vi "Export File - Rx Packet XML.vi"(4 "Rx Packet":T2 {"targetPriority" min=-2 max=16 step=1; "targetProcessor" min=-2 max=16 step=1; "Endianness" items=["big-endian"=0, "little-endian"=2]}, 6 "RootNode":refnum<k24>, 8 "error in (no error)":errorcluster, 9 "Rx Packet Header Data":T1, 11 "XmlDocument in":refnum<k24>) -> (0 "error out":errorcluster, 3 "XmlDocument out":refnum<k24>)   [LabVIEW 2019, in "UDP-Custom-Device System Explorer.lvlib"]
uses:
  UDP-Custom-Device System Explorer.lvlib
  System.Xml
  Types/XML - New/ImpExp - Rx Packet Data.ctl
  <vilib>/NI VeriStand/Custom Device API/Custom Device Item Info.ctl
  Shared/Types/Shared - Channel Data Type.ctl
  Shared/Types/Shared - Buffered.PacketInfo.ctl
  Shared/Types/Shared - Pointer Encoding.ctl
  Shared/Types/Shared - Receive Buffer Options.ctl
  Shared/Types/Shared - Transmit Buffer Options.ctl
  Shared/Types/Shared - New Data Options.ctl
  Shared/Types/Shared - Thread Management.ctl
  Types/XML - New/ImpExp - Packet Headers.ctl
  Shared/UDP-Custom-Device Shared.lvlib
  <vilib>/NI VeriStand/Custom Device API/Custom Device API.lvlib
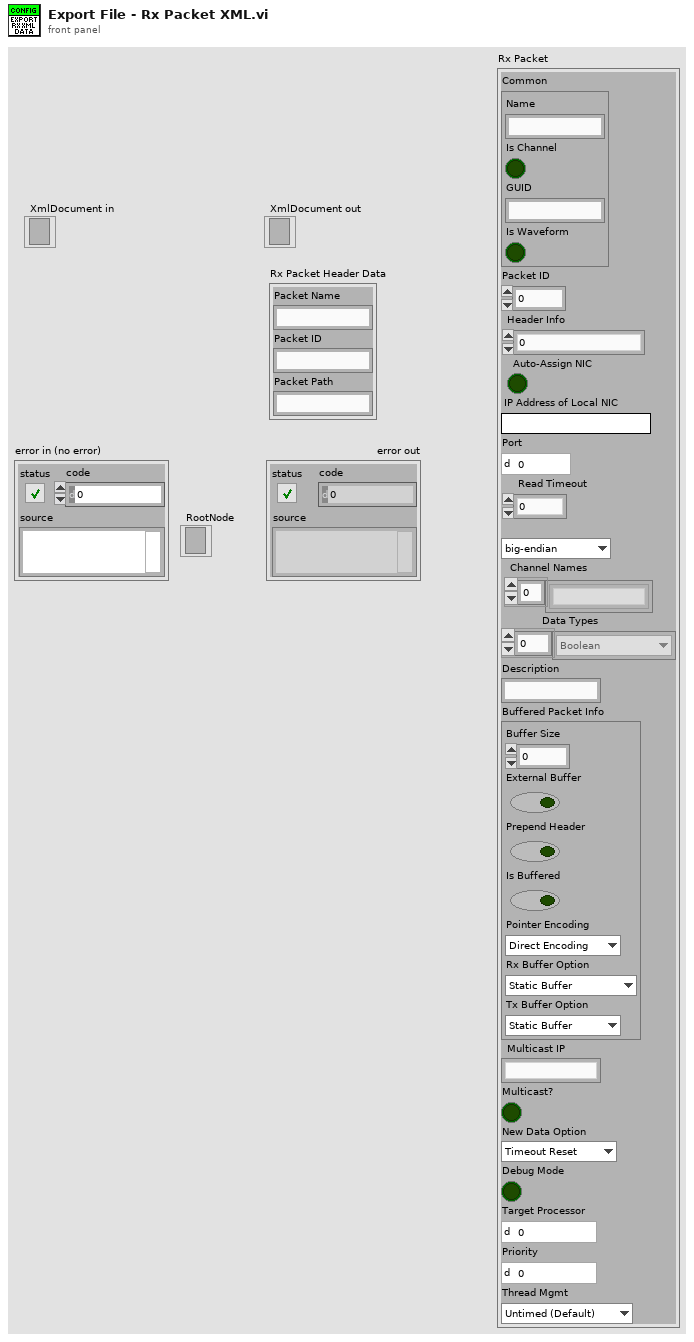
[diagram p1: front panel]
types:
  T1 = typedef "UDP-Custom-Device System Explorer.lvlib/ImpExp - Packet Headers.ctl" = cluster{"Packet Name":string, "Packet ID":string, "Packet Path":string}
  T2 = typedef "UDP-Custom-Device System Explorer.lvlib/ImpExp - Rx Packet Data.ctl" = cluster{"Common":T3, "Packet ID":i32, "Header Info":u32, "Auto-Assign NIC":bool, "IP Address of Local NIC":string, "Port":u16, "Read Timeout":i32, "Endianness":u16, "Channel Names":string[], "Data Types":T4[], "Description":string, "Buffered Packet Info":T5, "Multicast IP":string, "Multicast?":bool, "New Data Option":T9, "Debug Mode":bool, "targetProcessor":i8, "targetPriority":i16, "Thread Mgmt":T10}
  T3 = typedef "Custom Device API.lvlib/Custom Device Item Info.ctl" = cluster{"Name":string, "Is Channel":bool, "GUID":string, "Is Waveform":bool}
  T4 = typedef "UDP-Custom-Device Shared.lvlib/Shared - Channel Data Type.ctl" = enum16{"Boolean", "Single", "Double", "I8", "I16", "I32", "I64", "U8", "U16", "U32", "U64"}
  T5 = typedef "UDP-Custom-Device Shared.lvlib/Shared - Buffered.PacketInfo.ctl" = cluster{"Buffer Size":i32, "External Buffer":bool, "Prepend Header":bool, "Is Buffered":bool, "Pointer Encoding":T6, "Rx Buffer Option":T7, "Tx Buffer Option":T8}
  T6 = typedef "UDP-Custom-Device Shared.lvlib/Shared - Pointer Encoding.ctl" = enum16{"Direct Encoding", "Conversion Encoding"}
  T7 = typedef "UDP-Custom-Device Shared.lvlib/Shared - Receive Buffer Options.ctl" = enum16{"Static Buffer", "Circular Buffer", "Circular Buffer + Size", "Internal Cache", "Internal Cache + Size", "Ping Pong", "Ping Pong + Size"}
  T8 = typedef "UDP-Custom-Device Shared.lvlib/Shared - Transmit Buffer Options.ctl" = enum16{"Static Buffer", "FIFO Buffer", "FIFO Buffer + Port"}
  T9 = typedef "UDP-Custom-Device Shared.lvlib/Shared - New Data Options.ctl" = enum16{"Timeout Reset", "Counter"}
  T10 = typedef "UDP-Custom-Device Shared.lvlib/Shared - Thread Management.ctl" = enum16{"Untimed (Default)", "Timed (High Priority)"}
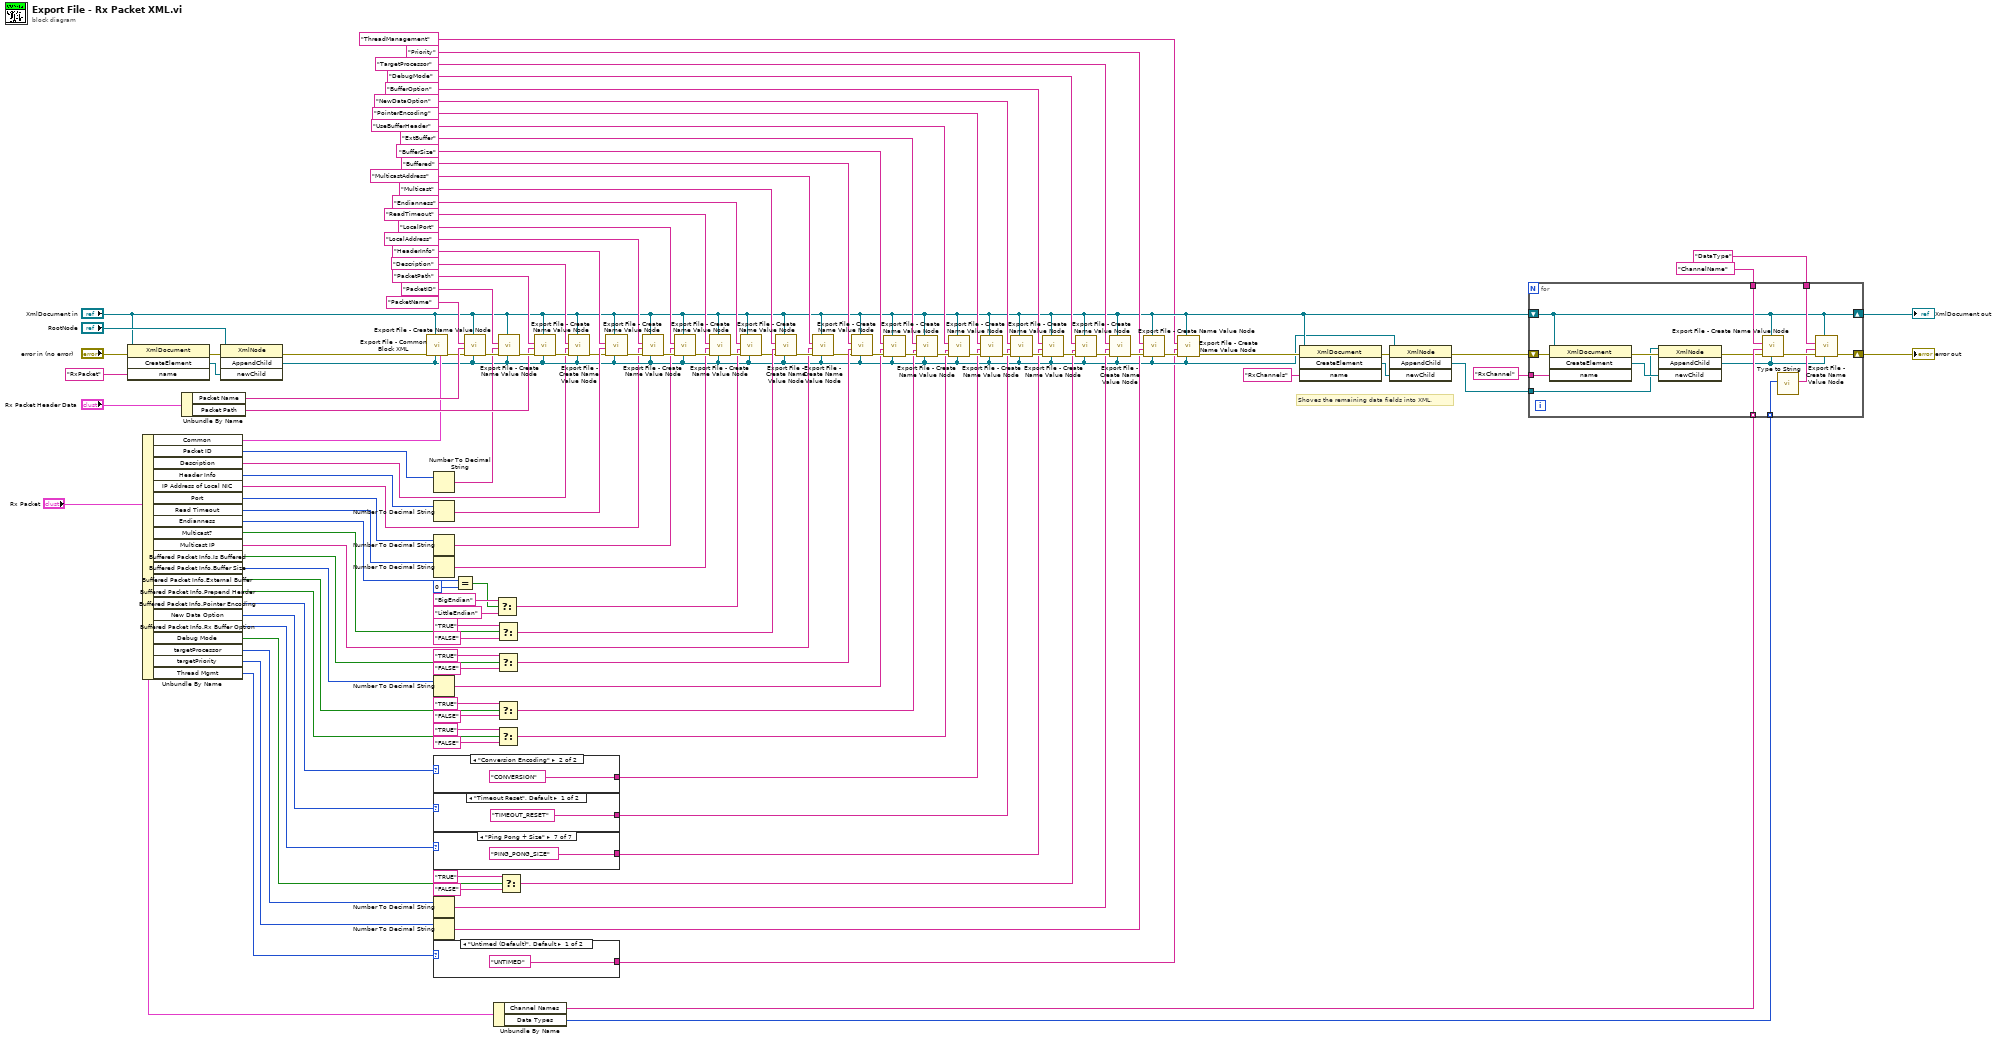
[diagram p0: block diagram]
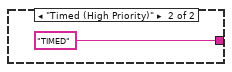
[diagram p2: hidden frame]
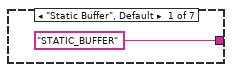
[diagram p3: hidden frame]
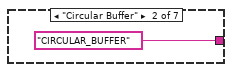
[diagram p4: hidden frame]
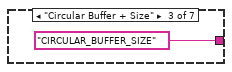
[diagram p5: hidden frame]
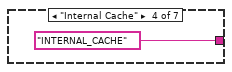
[diagram p6: hidden frame]
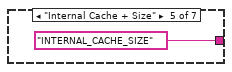
[diagram p7: hidden frame]
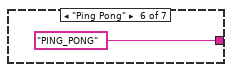
[diagram p8: hidden frame]
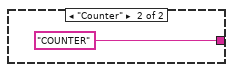
[diagram p9: hidden frame]
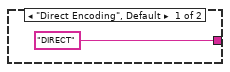
[diagram p10: hidden frame]
diagram:
  # "Shoves the remaining data fields into XML."
  n1 = invoke class="XmlDocument" method="CreateElement"(reference="XmlDocument in", error in="error in (no error)", "name"="RxPacket" ("Tag Name")) -> (error out=w111:errorcluster, "CreateElement"=w112:refnum<k24>)  [unwired: 1 in, 2 out]
  n2 = Unbundle By Name("Rx Packet") -> ("Common"=w106:T3, "Packet ID"=w83:i32, "Description"=w1:string, "Header Info"=w84:u32, "IP Address of Local NIC"=w2:string, "Port"=w94:u16, "Read Timeout"=w91:i32, "Endianness"=w89:u16, "Multicast?"=w43:bool, "Multicast IP"=w37:string, "Buffered Packet Info.Is Buffered"=w69:bool, "Buffered Packet Info.Buffer Size"=w70:i32, "Buffered Packet Info.External Buffer"=w68:bool, "Buffered Packet Info.Prepend Header"=w67:bool, "Buffered Packet Info.Pointer Encoding"=w35:T6, "New Data Option"=w29:T9, "Buffered Packet Info.Rx Buffer Option"=w27:T7, "Debug Mode"=w19:bool, "targetProcessor"=w13:i8, "targetPriority"=w12:i16, "Thread Mgmt"=w4:T10)
  n3 = Unbundle By Name("Rx Packet Header Data") -> ("Packet Name"=w115:string, "Packet Path"=w114:string)
  n4 = invoke class="XmlNode" method="AppendChild"(reference="RootNode", error in=w111, "newChild"=w112) -> (error out=w107:errorcluster, "AppendChild"=w6:refnum<k24>)  [unwired: 1 in, 2 out]
  n5 = call "Export File - Common Block XML.vi"("Common"=w106, "RootNode in"=w6, "XmlDocument in"="XmlDocument in", "error in (no error)"=w107) -> ("error out"=w110:errorcluster)  [unwired: 7 in]
  n6 = Number To Decimal String(number=w83) -> (decimal integer string=w82:string)  [unwired: 1 in]
  n7 = Number To Decimal String(number=w84) -> (decimal integer string=w98:string)  [unwired: 1 in]
  n8 = Number To Decimal String(number=w94) -> (decimal integer string=w93:string)  [unwired: 1 in]
  n9 = Number To Decimal String(number=w91) -> (decimal integer string=w90:string)  [unwired: 1 in]
  n10 = Number To Decimal String(number=w70) -> (decimal integer string=w61:string)  [unwired: 1 in]
  n11 = case shown="\"Conversion Encoding\"" w35 {
    tunnel: ["DIRECT" "CONVERSION"] -> w32
    frame "Direct Encoding", Default {
    }
    frame "Conversion Encoding" {
    }
  }
  n12 = case shown="\"Timeout Reset\", Default" w29 {
    tunnel: ["TIMEOUT_RESET" "COUNTER"] -> w28
    frame "Timeout Reset", Default {
    }
    frame "Counter" {
    }
  }
  n13 = case shown="\"Ping Pong + Size\"" w27 {
    tunnel: ["STATIC_BUFFER" "CIRCULAR_BUFFER" "CIRCULAR_BUFFER_SIZE" "INTERNAL_CACHE" "INTERNAL_CACHE_SIZE" "PING_PONG" "PING_PONG_SIZE"] -> w24
    frame "Static Buffer", Default {
    }
    frame "Circular Buffer" {
    }
    frame "Circular Buffer + Size" {
    }
    frame "Internal Cache" {
    }
    frame "Internal Cache + Size" {
    }
    frame "Ping Pong" {
    }
    frame "Ping Pong + Size" {
    }
  }
  n14 = Number To Decimal String(number=w13) -> (decimal integer string=w11:string)  [unwired: 1 in]
  n15 = Number To Decimal String(number=w12) -> (decimal integer string=w10:string)  [unwired: 1 in]
  n16 = case shown="\"Untimed (Default)\", Default" w4 {
    tunnel: ["UNTIMED" "TIMED"] -> w3
    frame "Untimed (Default)", Default {
    }
    frame "Timed (High Priority)" {
    }
  }
  n17 = Equal?(x=w89, y=u16 0) -> (x = y?=w79:bool)
  n18 = call "Export File - Create Name Value Node.vi"("RootNode in"=w6, "XmlDocument in"="XmlDocument in", "error in (no error)"=w110, "Value"=w115, "Name"="PacketName" ("Tag Name")) -> ("error out"=w121:errorcluster)  [unwired: 6 in]
  n19 = Unbundle By Name("Rx Packet") -> ("Channel Names"=w48:string[], "Data Types"=w47:T4[])
  n20 = Select(t="BigEndian", s=w79, f="LittleEndian") -> (s? t:f=w78:string)
  n21 = Select(t="TRUE", s=w43, f="FALSE") -> (s? t:f=w38:string)
  n22 = Select(t="TRUE", s=w69, f="FALSE") -> (s? t:f=w62:string)
  n23 = Select(t="TRUE", s=w68, f="FALSE") -> (s? t:f=w60:string)
  n24 = Select(t="TRUE", s=w67, f="FALSE") -> (s? t:f=w59:string)
  n25 = call "Export File - Create Name Value Node.vi"("RootNode in"=w6, "XmlDocument in"="XmlDocument in", "error in (no error)"=w121, "Value"=w82, "Name"="PacketID" ("Tag Name")) -> ("error out"=w120:errorcluster)  [unwired: 6 in]
  n26 = Select(t="TRUE", s=w19, f="FALSE") -> (s? t:f=w18:string)
  n27 = call "Export File - Create Name Value Node.vi"("RootNode in"=w6, "XmlDocument in"="XmlDocument in", "error in (no error)"=w120, "Value"=w114, "Name"="PacketPath" ("Tag Name")) -> ("error out"=w87:errorcluster)  [unwired: 6 in]
  n28 = call "Export File - Create Name Value Node.vi"("RootNode in"=w6, "XmlDocument in"="XmlDocument in", "error in (no error)"=w87, "Value"=w1, "Name"="Description" ("Tag Name")) -> ("error out"=w86:errorcluster)  [unwired: 6 in]
  n29 = call "Export File - Create Name Value Node.vi"("RootNode in"=w6, "XmlDocument in"="XmlDocument in", "error in (no error)"=w86, "Value"=w98, "Name"="HeaderInfo" ("Tag Name")) -> ("error out"=w105:errorcluster)  [unwired: 6 in]
  n30 = call "Export File - Create Name Value Node.vi"("RootNode in"=w6, "XmlDocument in"="XmlDocument in", "error in (no error)"=w105, "Value"=w2, "Name"="LocalAddress" ("Tag Name")) -> ("error out"=w104:errorcluster)  [unwired: 6 in]
  n31 = call "Export File - Create Name Value Node.vi"("RootNode in"=w6, "XmlDocument in"="XmlDocument in", "error in (no error)"=w104, "Value"=w93, "Name"="LocalPort" ("Tag Name")) -> ("error out"=w103:errorcluster)  [unwired: 6 in]
  n32 = call "Export File - Create Name Value Node.vi"("RootNode in"=w6, "XmlDocument in"="XmlDocument in", "error in (no error)"=w103, "Value"=w90, "Name"="ReadTimeout" ("Tag Name")) -> ("error out"=w102:errorcluster)  [unwired: 6 in]
  n33 = call "Export File - Create Name Value Node.vi"("RootNode in"=w6, "XmlDocument in"="XmlDocument in", "error in (no error)"=w102, "Value"=w78, "Name"="Endianness" ("Tag Name")) -> ("error out"=w36:errorcluster)  [unwired: 6 in]
  n34 = call "Export File - Create Name Value Node.vi"("RootNode in"=w6, "XmlDocument in"="XmlDocument in", "error in (no error)"=w36, "Value"=w38, "Name"="Multicast" ("Tag Name")) -> ("error out"=w42:errorcluster)  [unwired: 6 in]
  n35 = call "Export File - Create Name Value Node.vi"("RootNode in"=w6, "XmlDocument in"="XmlDocument in", "error in (no error)"=w42, "Value"=w37, "Name"="MulticastAddress" ("Tag Name")) -> ("error out"=w41:errorcluster)  [unwired: 6 in]
  n36 = call "Export File - Create Name Value Node.vi"("RootNode in"=w6, "XmlDocument in"="XmlDocument in", "error in (no error)"=w41, "Value"=w62, "Name"="Buffered" ("Tag Name")) -> ("error out"=w101:errorcluster)  [unwired: 6 in]
  n37 = call "Export File - Create Name Value Node.vi"("RootNode in"=w6, "XmlDocument in"="XmlDocument in", "error in (no error)"=w101, "Value"=w61, "Name"="BufferSize" ("Tag Name")) -> ("error out"=w100:errorcluster)  [unwired: 6 in]
  n38 = call "Export File - Create Name Value Node.vi"("RootNode in"=w6, "XmlDocument in"="XmlDocument in", "error in (no error)"=w100, "Value"=w60, "Name"="ExtBuffer" ("Tag Name")) -> ("error out"=w99:errorcluster)  [unwired: 6 in]
  n39 = call "Export File - Create Name Value Node.vi"("RootNode in"=w6, "XmlDocument in"="XmlDocument in", "error in (no error)"=w99, "Value"=w59, "Name"="UseBufferHeader" ("Tag Name")) -> ("error out"=w34:errorcluster)  [unwired: 6 in]
  n40 = call "Export File - Create Name Value Node.vi"("RootNode in"=w6, "XmlDocument in"="XmlDocument in", "error in (no error)"=w34, "Value"=w32, "Name"="PointerEncoding" ("Tag Name")) -> ("error out"=w31:errorcluster)  [unwired: 6 in]
  n41 = call "Export File - Create Name Value Node.vi"("RootNode in"=w6, "XmlDocument in"="XmlDocument in", "error in (no error)"=w31, "Value"=w28, "Name"="NewDataOption" ("Tag Name")) -> ("error out"=w26:errorcluster)  [unwired: 6 in]
  n42 = call "Export File - Create Name Value Node.vi"("RootNode in"=w6, "XmlDocument in"="XmlDocument in", "error in (no error)"=w26, "Value"=w24, "Name"="BufferOption" ("Tag Name")) -> ("error out"=w23:errorcluster)  [unwired: 6 in]
  n43 = call "Export File - Create Name Value Node.vi"("RootNode in"=w6, "XmlDocument in"="XmlDocument in", "error in (no error)"=w23, "Value"=w18, "Name"="DebugMode" ("Tag Name")) -> ("error out"=w17:errorcluster)  [unwired: 6 in]
  n44 = call "Export File - Create Name Value Node.vi"("RootNode in"=w6, "XmlDocument in"="XmlDocument in", "error in (no error)"=w17, "Value"=w11, "Name"="TargetProcessor" ("Tag Name")) -> ("error out"=w16:errorcluster)  [unwired: 6 in]
  n45 = call "Export File - Create Name Value Node.vi"("RootNode in"=w6, "XmlDocument in"="XmlDocument in", "error in (no error)"=w16, "Value"=w10, "Name"="Priority" ("Tag Name")) -> ("error out"=w9:errorcluster)  [unwired: 6 in]
  n46 = call "Export File - Create Name Value Node.vi"("RootNode in"=w6, "XmlDocument in"="XmlDocument in", "error in (no error)"=w9, "Value"=w3, "Name"="ThreadManagement" ("Tag Name")) -> ("error out"=w8:errorcluster)  [unwired: 6 in]
  n47 = invoke class="XmlDocument" method="CreateElement"(reference="XmlDocument in", error in=w8, "name"="RxChannels" ("Tag Name")) -> (error out=w55:errorcluster, "CreateElement"=w57:refnum<k24>)  [unwired: 1 in, 2 out]
  n48 = invoke class="XmlNode" method="AppendChild"(reference=w6, error in=w55, "newChild"=w57) -> (error out=w54:errorcluster, "AppendChild"=w52:refnum<k24>)  [unwired: 1 in, 2 out]
  n49 = for {
    shift-right: [w148] -> w53
    shift-left: w54 -> [w140]
    tunnel: w52 -> [w137]
    shift-right: [w141] -> w51
    shift-left: "XmlDocument in" -> [w141]
    tunnel: "ChannelName" ("Tag Name") -> [w147]
    tunnel: "DataType" ("Tag Name") -> [w146]
    tunnel: w48 -> [w145] mode=indexing
    tunnel: w47 -> [w144] mode=indexing
    tunnel: "RxChannel" ("Tag Name") -> [w138]
    n50 = invoke class="XmlDocument" method="CreateElement"(reference=w141, error in=w140, "name"=w138) -> (error out=w139:errorcluster, "CreateElement"=w142:refnum<k24>)  [unwired: 1 in, 2 out]
    n51 = invoke class="XmlNode" method="AppendChild"(reference=w137, error in=w139, "newChild"=w142) -> (error out=w135:errorcluster, "AppendChild"=w136:refnum<k24>)  [unwired: 1 in, 2 out]
    n52 = call "Export File - Create Name Value Node.vi"("RootNode in"=w136, "XmlDocument in"=w141, "error in (no error)"=w135, "Value"=w145, "Name"=w147) -> ("error out"=w149:errorcluster)  [unwired: 6 in]
    n53 = call "Type to String.vi"("Data Type"=w144) -> ("String Type"=w143:string)  [unwired: 10 in]
    n54 = call "Export File - Create Name Value Node.vi"("RootNode in"=w136, "XmlDocument in"=w141, "error in (no error)"=w149, "Value"=w143, "Name"=w146) -> ("error out"=w148:errorcluster)  [unwired: 6 in]
  }
  "error out" <- w53
  "XmlDocument out" <- w51
